vi "RW Controls INI.vi"(0 "PIinfo In":T2(array[cluster]), 1 "Filepath":path, 2 "Read (F)":bool, 5 "CutoffArray In":cluster{"MidCutoff":dbl, "CloseCutoff":dbl}[](array[cluster]), 7 "FFinfo In":T1(array[cluster]), 9 "LimitsArray In":cluster{"Step":dbl, "Max":dbl, "Min":dbl}[](array[cluster]), 11 "Error In":errorcluster) -> (4 "PIinfo Out":T2(array[cluster]), 6 "CutoffArray Out":cluster{"MidCutoff":dbl, "CloseCutoff":dbl}[](array[cluster]), 8 "FFinfo Out":T1(array[cluster]), 10 "LimitsArray Out":cluster{"Step":dbl, "Max":dbl, "Min":dbl}[](array[cluster]), 15 "Error Out":errorcluster)   [LabVIEW 2013]
uses:
  <vilib>/Utility/config.llb/NI_LVConfig.lvlib
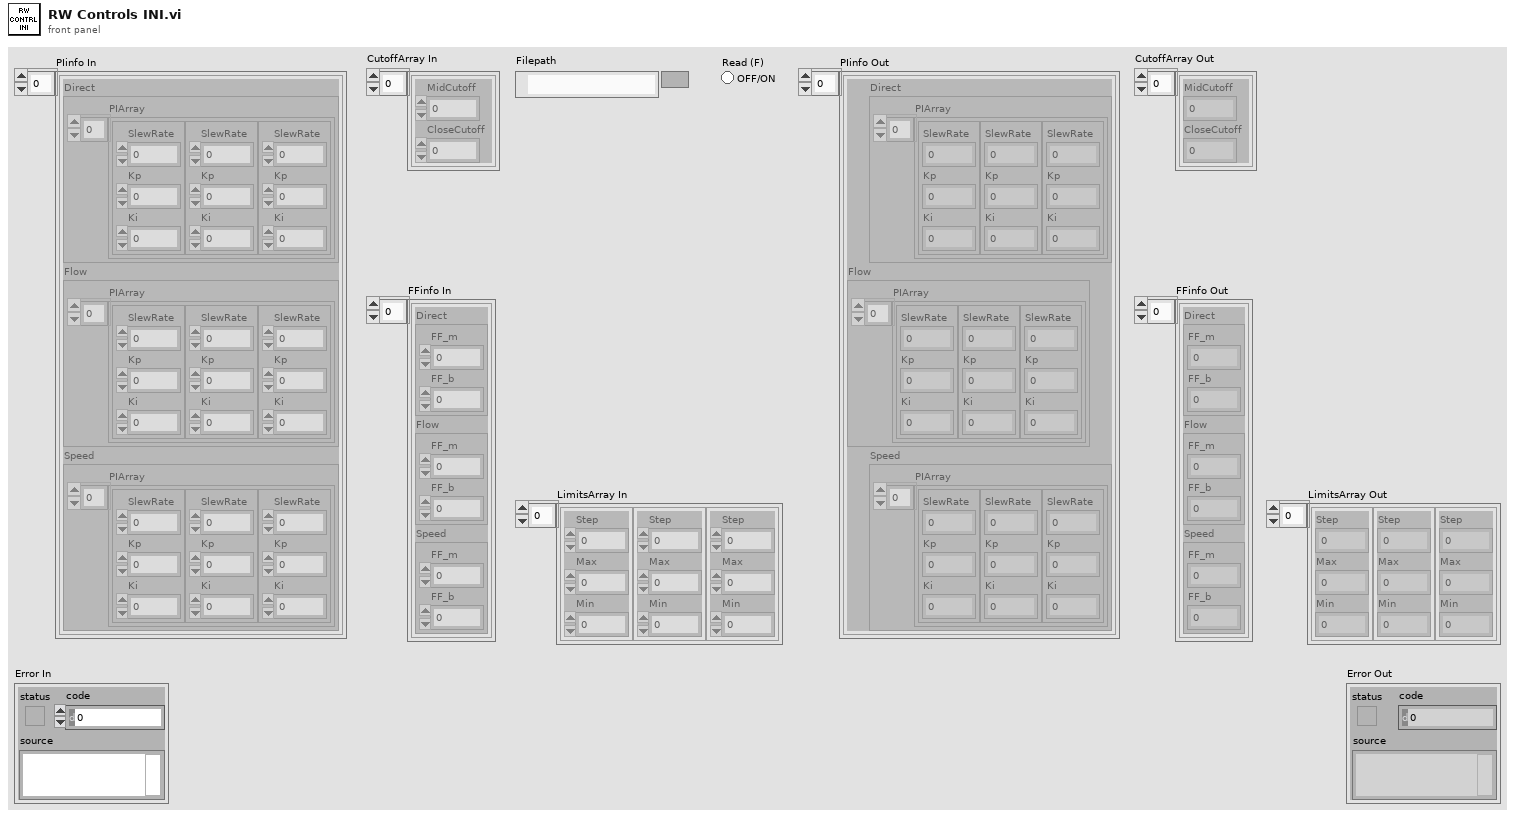
[diagram p1: front panel]
types:
  T1 = cluster{"Direct":cluster{"FF_m":dbl, "FF_b":dbl}, "Flow":cluster{"FF_m":dbl, "FF_b":dbl}, "Speed":cluster{"FF_m":dbl, "FF_b":dbl}}[]
  T2 = cluster{"Direct":cluster{"PIArray":cluster{"SlewRate":dbl, "Kp":dbl, "Ki":dbl}[]}, "Flow":cluster{"PIArray":cluster{"SlewRate":dbl, "Kp":dbl, "Ki":dbl}[]}, "Speed":cluster{"PIArray":cluster{"SlewRate":dbl, "Kp":dbl, "Ki":dbl}[]}}[]
  T3 = typedef "NI_LVConfig.lvlib/Config Data RefNum.ctl" = refnum<k1>
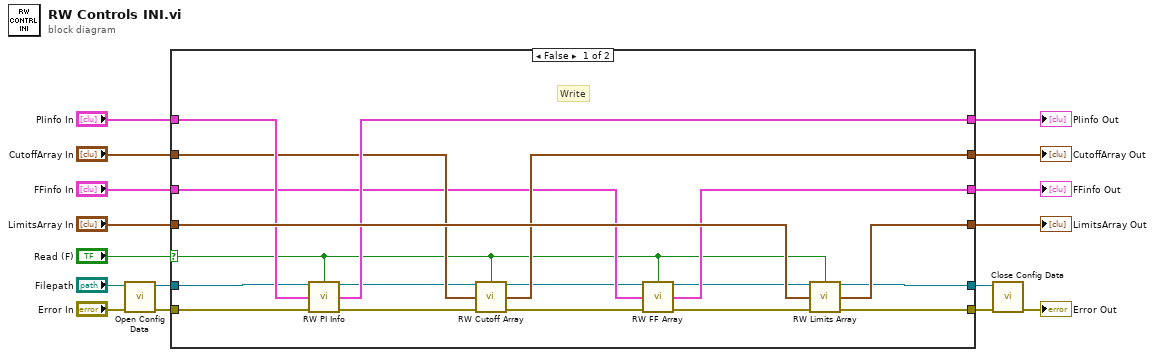
[diagram p0: block diagram]
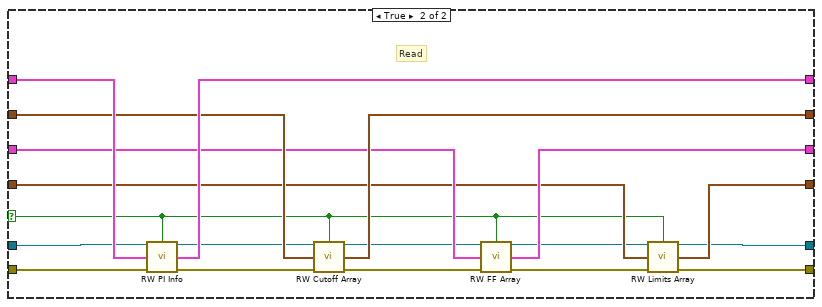
[diagram p2: hidden frame]
diagram:
  n1 = call <vilib>:"Open Config Data.vi"("error in (no error)"="Error In", "configuration file path"="Filepath") -> ("error out"=w12:errorcluster, "refnum"=w11:T3)  [unwired: 7 in, 1 out]
  n2 = case shown="False" "Read (F)" {
    selector: "Read (F)" -> [w22 w41]
    tunnel: w12 -> [w35 w54]
    tunnel: w11 -> [w21 w40]
    tunnel: [w31 w50] -> w10
    tunnel: "PIinfo In" -> [w25 w49]
    tunnel: "CutoffArray In" -> [w24 w47]
    tunnel: "FFinfo In" -> [w23 w45]
    tunnel: "LimitsArray In" -> [w30 w43]
    tunnel: [w29 w42] -> w5
    tunnel: [w28 w44] -> w4
    tunnel: [w27 w46] -> w3
    tunnel: [w26 w48] -> w2
    tunnel: [w17 w36] -> w1
    frame False {
      # "Write"
      n3 = call "RW PI Info.vi"("Refnum In"=w21, "Read (F)"=w22, "PIinfo In"=w25, "Error In"=w35) -> ("Refnum Out"=w20:T3, "PIinfo Out"=w26:T2, "Error Out"=w34:errorcluster)  [unwired: 9 in]
      n4 = call "RW Cutoff Array.vi"("Refnum In"=w20, "Read (F)"=w22, "CutoffArray In"=w24, "Error In"=w34) -> ("Refnum Out"=w19:T3, "CutoffArray Out"=w27:cluster{"MidCutoff":dbl, "CloseCutoff":dbl}[], "Error Out"=w33:errorcluster)  [unwired: 9 in]
      n5 = call "RW FF Array.vi"("Refnum In"=w19, "Read (F)"=w22, "FFinfo In"=w23, "Error In"=w33) -> ("Refnum Out"=w18:T3, "FFinfo Out"=w28:T1, "Error Out"=w32:errorcluster)  [unwired: 9 in]
      n6 = call "RW Limits Array.vi"("Refnum In"=w18, "Read (F)"=w22, "LimitsArray In"=w30, "Error In"=w32) -> ("Refnum Out"=w17:T3, "LimitsArray Out"=w29:cluster{"Step":dbl, "Max":dbl, "Min":dbl}[], "Error Out"=w31:errorcluster)  [unwired: 9 in]
    }
    frame True {
      # "Read"
      n7 = call "RW PI Info.vi"("Refnum In"=w40, "Read (F)"=w41, "PIinfo In"=w49, "Error In"=w54) -> ("Refnum Out"=w39:T3, "PIinfo Out"=w48:T2, "Error Out"=w53:errorcluster)  [unwired: 9 in]
      n8 = call "RW Cutoff Array.vi"("Refnum In"=w39, "Read (F)"=w41, "CutoffArray In"=w47, "Error In"=w53) -> ("Refnum Out"=w38:T3, "CutoffArray Out"=w46:cluster{"MidCutoff":dbl, "CloseCutoff":dbl}[], "Error Out"=w52:errorcluster)  [unwired: 9 in]
      n9 = call "RW FF Array.vi"("Refnum In"=w38, "Read (F)"=w41, "FFinfo In"=w45, "Error In"=w52) -> ("Refnum Out"=w37:T3, "FFinfo Out"=w44:T1, "Error Out"=w51:errorcluster)  [unwired: 9 in]
      n10 = call "RW Limits Array.vi"("Refnum In"=w37, "Read (F)"=w41, "LimitsArray In"=w43, "Error In"=w51) -> ("Refnum Out"=w36:T3, "LimitsArray Out"=w42:cluster{"Step":dbl, "Max":dbl, "Min":dbl}[], "Error Out"=w50:errorcluster)  [unwired: 9 in]
    }
  }
  "PIinfo Out" <- w2
  "CutoffArray Out" <- w3
  "FFinfo Out" <- w4
  "LimitsArray Out" <- w5
  n11 = call <vilib>:"Close Config Data.vi"("error in (no error)"=w10, "refnum"=w1) -> ("error out"=→"Error Out":errorcluster)  [unwired: 8 in, 1 out]
